vi "OAT Torsional Vibration (Digital Tacho) (Even-Angle) (N Ch - N Settings).vi"(0 "digital tacho info":T7[](array[typedef]), 2 "pulse/revolution (1)":i32[](array[numeric]) min=1, 4 "torsional vibration units":enum16{"RPM", "deg/s", "rad/s"}(ring), 5 "error in (no error)":errorcluster, 8 "reset? (F)":bool) -> (14 "even-angle torsional vibration signals":cluster{"r0":dbl, "dr":dbl, "Y":dbl[]}[](array[cluster]) {"r0" format="%.2p"; "dr" format="%.2p"; "Y" format="%.2f"}, 15 "even-angle channel info":T3[](array[typedef]) {"channel info"."pregain" format="%.2f"; "channel info"."weighting filter" items=["Linear", "A-weighting", "B-weighting", "C-weighting", "ITU-R 468-4", "Dolby", "CCITT", "C-message", "Wb", "Wc", "Wd", "We", "Wf", "Wh", "Wj", "Wk", "Wm", "AES17 20 kHz lowpass", "AES17 40 kHz lowpass", "AES17 20 kHz highpass", "AES17 40 kHz highpass"]; "channel info"."dB reference" format="%^.1e"; "channel info"."engineering units" items=["custom..."=0, "V"=1, "A"=21, "C"=30, "pC"=31, "s"=32, "-"=29, "Pa"=2, "N"=20, "g"=3, "m/s^2"=4, "m/s"=5, "m"=6, "mm/s"=12, "mm"=13, "micron/s"=14, "micron"=15, "in/s^2"=7, "in/s"=8, "in"=9, "mil/s"=10, "mil"=11, "rad/s^2"=16, "rad/s"=17, "rad"=18, "deg/s^2"=26, "deg/s"=27, "deg"=28, "RPM"=22, "cycle/s^2"=23, "Hz"=24, "cycle"=25, "strain"=19]; "channel info"."sensor sensitivity" format="%#_5f"}, 16 "speed profiles":T2[](array[typedef]) {"speed [RPM]" format="%.2f"; "time [s]" format="%.2f"}, 17 "position info":T1[](array[typedef]), 18 "unit labels":string[](array[string]), 19 "error out":errorcluster)   [LabVIEW 2017, in "SoundVib_Torsional.lvlib"]
doc: "Calculates torsional vibration signals from digital tachometer signals. This VI can return torsional vibration signals as either waveform signals or even-angle signals. Wire data to the <B>digital tacho info</B> input to determine the polymorphic instance to use or manually select the instance."
uses:
  <vilib>/addons/Sound and Vibration/Order Analysis/Torsional Vibration/SoundVib_Torsional.lvlib
  <vilib>/addons/Sound and Vibration/Order Analysis/Tach Process/SubVIs/digital tach info.ctl
  <vilib>/addons/_NISVFA/_Shared subVIs/Controls/svc_Resampled Channel Info.ctl
  <vilib>/addons/_NISVFA/_Shared subVIs/Controls/svc_Channel Info.ctl
  <vilib>/addons/_NISVFA/_Shared subVIs/Controls/svc_Engineering Units Text Ring.ctl
  <vilib>/addons/_NISVFA/_Shared subVIs/Controls/svc_Weighting Filter Text Ring.ctl
  <vilib>/addons/Sound and Vibration/Order Analysis/Tach Process/SubVIs/speed profile.ctl
  <vilib>/addons/Sound and Vibration/Order Analysis/Misc/OAT Position Info.ctl
  <vilib>/addons/Sound and Vibration/Order Analysis/Tach Process/SoundVib_TachProcess.lvlib
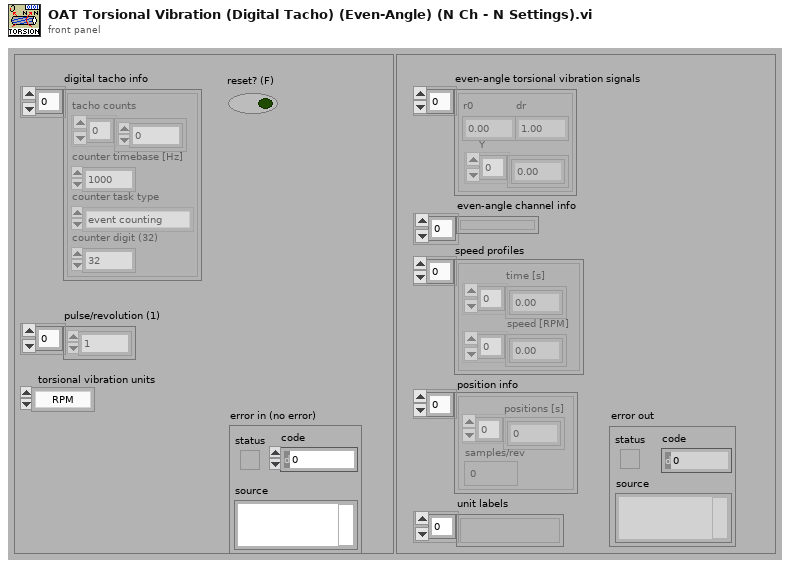
[diagram p1: front panel]
types:
  T1 = typedef "OAT Position Info.ctl" = cluster{"positions [s]":dbl[], "samples/rev":dbl}
  T2 = typedef "SoundVib_TachProcess.lvlib/speed profile.ctl" = cluster{"time [s]":dbl[], "speed [RPM]":dbl[]}
  T3 = typedef "svc_Resampled Channel Info.ctl" = cluster{"channel name":string, "description":string, " channel info":T4}
  T4 = typedef "svc_Channel Info.ctl" = cluster{"sensor sensitivity":dbl, "engineering units":T5, "dB reference":dbl, "custom label":string, "weighting filter":T6, "pregain":dbl}
  T5 = typedef "svc_Engineering Units Text Ring.ctl" = u16
  T6 = typedef "svc_Weighting Filter Text Ring.ctl" = u16
  T7 = typedef "SoundVib_TachProcess.lvlib/digital tach info.ctl" = cluster{"tacho counts":i64[], "counter timebase [Hz]":dbl, "counter task type":enum16{"period measurement", "event counting"}, "counter digit (32)":i32}
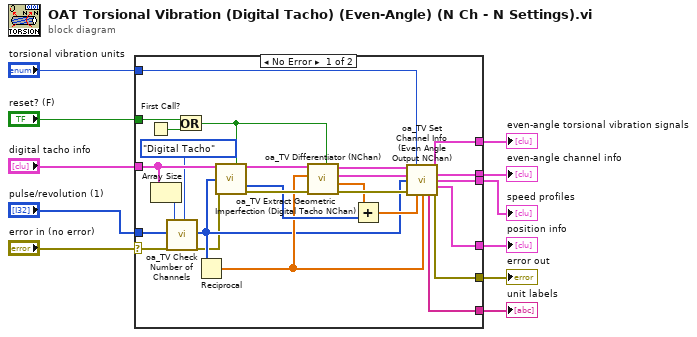
[diagram p0: block diagram]
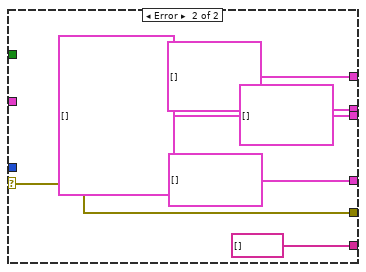
[diagram p2: hidden frame]
diagram:
  n1 = case shown="No Error" "error in (no error)" {
    selector: "error in (no error)" -> [w18 w43]
    tunnel: "reset? (F)" -> [w34 _]
    tunnel: "digital tacho info" -> [w15 _]
    tunnel: "pulse/revolution (1)" -> [w16 _]
    tunnel: "torsional vibration units" -> [w24 _]
    tunnel: [w27 T3[] [] ("even-angle channel info")] -> w6
    tunnel: [w26 cluster{"r0":dbl, "dr":dbl, "Y":dbl[]}[] [] ("even-angle torsional vibration")] -> w5
    tunnel: [w30 w43] -> w8
    tunnel: [w23 string[] [] ("unit labels")] -> w3
    tunnel: [w22 T2[] [] ("speed profiles")] -> w2
    tunnel: [w21 T1[] [] ("position info")] -> w1
    frame No Error {
      n2 = First Call?() -> (First Call?: T/F=w35:bool)
      n3 = Array Size(array=w15) -> (size(s)=w14:i32)
      n4 = call <vilib>:"oa_TV Check Number of Channels.vi"("pulse/revolution (1)"=w16, "error in (no error)"=w18, "channel number"=w14, "tacho selection"=enum16{"Analog Tacho", "Digital Tacho"}."Digital Tacho") -> ("pulse/revolution out"=w19:i32[], "error out"=w17:errorcluster)  [unwired: 9 in, 5 out]
      n5 = Or(x=w34, y=w35) -> (x .or. y?=w32:bool)
      n6 = Reciprocal(x=w19) -> (1/x=w29:dbl[])
      n7 = call <vilib>:"oa_TV Extract Geometric Imperfection (Digital Tacho NChan).vi"("digital tacho info"=w15, "reset? (F)"=w32, "pulse/revolution"=w19, "error in (no error)"=w17) -> ("pulse positions"=w33:cluster{dbl[]}[], "revulotion index"=w36:i32[], "error out"=w37:errorcluster)  [unwired: 8 in, 1 out]
      n8 = call <vilib>:"oa_TV Differentiator (NChan).vi"("reset? (False)"=w32, "error in (no error)"=w37, "delta X"=w29, "Y[n]"=w33) -> ("error out"=w31:errorcluster, "Delay"=w12:dbl[], "X[n]"=w20:cluster{dbl[]}[], "dY[n]/dX[n]"=w25:cluster{dbl[]}[])  [unwired: 4 in]
      n9 = Add(x=w12, y=w36) -> (x+y=w28:dbl[])
      n10 = call <vilib>:"oa_TV Set Channel Info (Even Angle Output NChan).vi"("seconds/revolution"=w25, "torisional vibration unit (RPM)"=w24, "pulse positions"=w20, "pulse/revolution (1)"=w19, "error in (no error)"=w31, "r0"=w28, "dr"=w29) -> ("even-angle torsional vibration"=w26:cluster{"r0":dbl, "dr":dbl, "Y":dbl[]}[], "even-angle channel info"=w27:T3[], "speed profiles"=w22:T2[], "position info"=w21:T1[], "unit labels"=w23:string[], "error out"=w30:errorcluster)  [unwired: 3 in]
    }
    frame Error {
    }
  }
  "error out" <- w8
  "even-angle channel info" <- w6
  "even-angle torsional vibration signals" <- w5
  "unit labels" <- w3
  "speed profiles" <- w2
  "position info" <- w1
